vi "Combo_While_For_Loop.vi"() -> ()   [LabVIEW 2020]
panel:
  out "stop_iteration":dbl
  in  "max_iter":i32
  in  "stop":bool
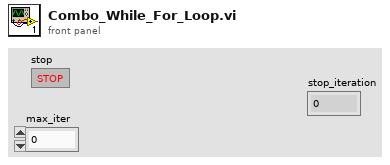
[diagram p1: front panel]
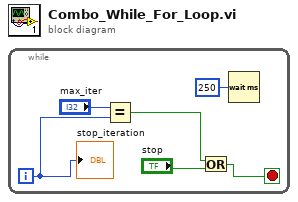
[diagram p0: block diagram]
diagram:
  n1 = while {
    i -> [w2]
    stop <- w6 stop-if-true
    n2 = Equal?(x="max_iter", y=w2) -> (x = y?=w4:bool)
    n3 = Or(x=w4, y="stop") -> (x .or. y?=w6:bool)
    n4 = Wait (ms)(milliseconds to wait=u32 250) -> ()  [unwired: 1 out]
    "stop_iteration" <- w2
  }
